vi "Power Peak Calibration.vi"() -> ()   [LabVIEW 2013]
uses:
  <vilib>/Analysis/NI_AALPro.lvlib
panel:
  in  "Acquire Data":bool
  out "df":dbl
  out "Calibration Data":dbl[](array[numeric])
  in  "Record Power Peak":bool
  out "Power Peak (V_{rms}^2)":dbl
  out "Spectrum Plot":cluster{dbl, "df":dbl, "Spectrum out":dbl[]}(graph)={0.0, "df"=976.5625, "Spectrum out"=[-15.845905781941731, -43.915142224307615, -49.190152957598016, -53.852042141976526, -56.401103239588394, -57.085019943821614, -57.42779024840779, -57.35398394101817, -56.62922799689663, -55.89570951726039, -56.17500389904336, -56.658091219147195, -57.96434809011062, -59.59705407171775, -60.67339237533791, -61.360791233190774, -62.26267752184724, -63.423104999089006, -63.73866172675654, -64.18018519332178, -64.68423775328336, -64.98272548894641, -64.65310396761447, -64.57730161736126, -64.6005007874894, -64.12943876516434, -64.40965139054964, -64.48190909962165, -64.18589412754218, -64.42687756848638, -64.73568364963023, -65.28016436445176, -65.51147244197554, -65.98403978636362, -66.34146853538246, -66.55039985238902, -67.06053323082511, -67.74164293441598, -67.93985420802743, -68.61366318004022, -68.72894399366066, -68.87062306002007, -69.25800759395273, -69.1836018440649, -69.6828981066074, -70.13235629974473, -70.02165546204415, -70.33805295925532, -70.33684508822006, -70.7747643357369, -70.92095605059647, -70.96159422425444, -71.51578558675507, -71.41022976627563, -71.51054007786686, -71.70594752739161, -71.89852623371247, -72.25001369052693, -72.05827807939693, -72.39722220210967, -72.26810938379876, -72.41633072401957, -72.89508447023017, -72.99611346447384, -72.86737450753068, -73.0319650267352, -73.4268723195781, -73.65485289175722, -73.76856016219259, -74.38259001523501, -74.49537543116152, -74.74289986108654, -74.52927345921171, -74.90899995658931, -75.12881029655497, -75.14682651299673, -76.04632955612527, -75.94928207346015, -75.99537357070861, -76.4528123167457, -76.58018971613478, -76.85262666813362, -76.94211368376116, -77.18033274801466, -77.34416946182976, -77.97653501905563, -78.08882898139076, -77.75504318146395, -78.61320071718298, -78.70255681878588, -78.89431147000928, -79.14802147917631, -79.24488934190079, -79.65778031243343, -79.75057207068667, -79.77429060312991, -80.22466006530694, -80.68765140609128, -80.74976372106957, -81.0940546603702, -81.06408506915871, -81.82084451213092, -81.88988589649128, -81.84353327749841, -82.71246581831555, -82.51089752593228, -82.76564863813098, -83.37330766537886, -83.57000868373369, -84.207392955926, -83.969059548894, -83.78119345015493, -84.68397306775822, -85.0123761871565, -85.04032792293864, -85.23566564306427, -85.49339332769287, -86.10740873526836, -86.30750461634167, -86.4954000769498, -86.58840326479293, -86.89617522722962, -87.03534322616281, -87.46765008133713, -87.51609655554547, -88.10480512426382, -88.53915071524821, -88.19089444702308, -88.76142323860263, -88.71484736501934, -89.39078167881094, -89.1390929539335, -89.73983451982647, -89.43411209172332, -90.07683547720683, -89.84084792738655, -90.03935645658841, -90.50074846778033, -90.62364106944639, -90.51858213646457, -90.77967673354854, -90.93487931797472, -90.49480094125931, -90.3356032916364, -91.24246400073463, -91.48972525529442, -91.56992962340016, -91.76393867194281, -92.24132938539142, -91.75033976436218, -92.23161782472576, -87.81832550071526, -91.95848559189331, -92.41846454494608, -92.44911534680506, -92.40717315350687, -92.64568182466519, -92.57261319696957, -92.68207058954437, -92.9414768787689, -92.99508291320579, -92.867293420003, -92.94829912779514, -93.22977946462234, -93.1496226108207, -93.32130652503764, -93.23714576357534, -92.71904125124473, -93.18861501311126, -93.34592185157314, -93.45645354610178, -93.29578779965661, -93.3961297071871, -93.52984447013718, -92.02818183792024, -92.17337335281373, -93.28573212068224, -93.4340403695752, -93.84898362415335, -93.8581389607782, -93.89732009520142, -93.8717074429978, -93.55264052897613, -93.50847613972101, -94.08331357574471, -94.07085225312551, -94.12661608080454, -94.3287445314006, -94.21766199449495, -94.27011202232808, -93.74524014468926, -94.35069940715115, -94.57610154940247, -94.52140154491451, -94.506512103288, -94.56804830787351, -94.49032013599088, -94.46360025059532, -94.28632692138267, -94.49959977802484, -94.50646018472031, -94.40554926428291, -94.68078780859665, -94.64664127985617, -94.66194886677796, -94.47957139621263, -93.31930218448838, -91.90550929382852, -94.34111457198259, -94.68074039683111, -94.79277504034081, -94.67994321030025, -94.86846988585798, -94.59982729948628, -94.07756932717759, -93.94330857800993, -94.30027374612484, -94.96329133863675, -94.77334352200275, -95.17028193906157, -95.21627296027212, -94.89033645488158, -95.20261401452001, -94.7704132670353, -95.42628192610192, -95.15102974391041, -95.18733765508992, -95.14908122444831, -95.4464140437162, -95.42528161153442, -94.48555734817637, -95.1993983585333, -95.39889184869536, -95.4903325691213, -95.48979359017684, -95.48200245883402, -95.49936365987897, -95.24916272786852, -91.91217566611354, -94.47496647183172, -95.27773576498515, -95.62838774635402, -95.71895141030696, -95.88390829882444, -95.56255178116972, -95.56813843723248, -95.07076550467647, -95.41001727617747, -95.58615607679087, -95.74834461273437, -95.77760596931367, -95.97902444733214, -95.94618628531285, -96.125407389205, -96.05556462687056, -95.63456098032873, -95.85612018930411, -95.80426046264252, -95.85838083397036, -95.70135694128692, -95.92486020964407, -95.77151462988817, -95.56348235993723, -95.63278256966903, -95.92343511351353, -95.84676472701682, -95.98333279604728, -96.25747326594166, -95.91741144469422, -95.36123720048207, -93.53184100084428, -95.92088328158893, -95.67059250119598, -96.08314273525487, -96.08815002286863, -96.22857738603786, -95.79857795122776, -95.73640081941579, -87.83199015388689, -95.89330062152945, -96.38888519003386, -96.39583952467083, -96.48390492192655, -96.61453120154768, -96.67350640699806, -96.56146072576644, -96.27150366452624, -96.59490502386653, -96.42327820826156, -96.49183302613625, -96.53913950676514, -96.49314016260925, -96.23812751552953, -95.8866021994261, -95.54556448224449, -96.45802589344208, -96.7081588901148, -96.34268723583261, -96.5775070247212, -96.0158615492137, -95.60991718375256, -92.98295890874621, -93.1175643950674, -95.48928276599159, -96.22343360123936, -96.58719806894042, -96.25366695891285, -96.70869216556476, -96.75664104310033, -95.99058593639634, -94.64288633299653, -96.39354296370634, -96.72512038071808, -96.89323897924083, -97.16294983631505, -96.99550829692208, -97.07580684762681, -97.05727223406919, -96.81028630212607, -97.00924445063612, -96.93954724005931, -96.910905559072, -97.25053999912566, -97.09809186624064, -96.99480693304544, -96.75674825164693, -96.71418496792745, -97.01481312025051, -96.98148452558607, -97.01830796226021, -96.69339813471524, -96.59361393554506, -96.4309846912819, -94.38407178672736, -92.50436488753007, -96.01557282796318, -96.39356474689868, -97.01610959436871, -97.05636935662201, -96.94226548253532, -96.0803835936364, -94.55887738493533, -94.20134587085661, -95.49518187885134, -96.66382783262259, -96.86250971219577, -97.00560385732297, -96.96730073141048, -97.0953639128831, -96.89780822210325, -96.48712240274082, -96.7856155647513, -96.72125010071417, -96.58394972410399, -96.6221299103751, -96.66884759315269, -96.73433925619264, -96.33613482351356, -96.89289999301926, -96.03898417460942, -97.09920512469947, -96.97039713471543, -96.67214133783074, -96.78650672809556, -95.9112797853549, -88.64340678313235, -95.24547674087896, -96.68477510092077, -97.26506755337493, -97.1141231148176, -97.2139546520637, -97.30526535922769, -97.18621986933206, -94.2064163293791, -96.39143663947267, -97.2802323889613, -97.54892117980299, -97.36965609295105, -97.26059900417418, -97.11769961105392, -96.61078438140439, -97.23469909611896, -97.7011904395048, -97.39540003198924, -97.31676145868914, -97.49636186951997, -97.19736596978883, -97.06772766971199, -96.63770097352807, -96.53253764690933, -96.24702084266804, -96.41431118366324, -96.0911845626953, -95.83696385570606, -95.78547289086474, -95.20587090233619, -94.14965366487957, -91.98394335062423, -94.42258288009647, -94.86573505676839, -95.20179207612364, -95.78589887823911, -96.02483899744861, -96.3232417400719, -94.37664270069325, -84.63776042475754, -95.90833150645543, -96.85168271545405, -96.94917553463841, -97.25201393296331, -97.19803469804113, -97.44067231757063, -97.28856434493133, -96.28089076443857, -97.40157405797581, -97.29153510147472, -97.60517422678114, -97.57431936262054, -97.3721504279831, -97.53879903587708, -96.19909166372716, -96.25534829018159, -97.09750465448909, -97.00543625791937, -97.15095351396809, -96.58677119756445, -95.86194320630636, -93.96685771994126, -90.41654167200038, -91.0693693812922, -94.9513584929577, -96.28027049834664, -96.94590502670485, -96.94649852135676, -96.93113649614565, -96.56082193420788, -95.07817706510154, -93.86060076780025, -96.52071349387154, -97.21608851333141, -97.41488438212835, -97.46100333688378, -97.54199390581512, -97.58802567652239, -97.73748653957938, -97.41143723707317, -97.64500942619026, -97.74567328179786, -97.31304599093758, -97.68415263166796, -97.47817511849203, -97.48054466789846, -97.04145721392551, -97.13368056999023, -97.02339838743785, -97.32646604511258, -97.29690558109404, -97.39432260133225, -96.5389671686748, -96.36745891004183, -93.32306114208308, -93.52279253865957, -96.06301720725452, -96.99679379652507, -97.22296553195883, -96.7803464077598, -96.17262512321993, -94.41741314352049, -90.69349735405582, -90.30864158287707, -93.60468105114984, -95.72116646020368, -96.72892404876248, -97.29206802349279, -97.33409428132504, -96.89003477779283, -96.65097311154193, -95.67336679796946, -97.35096090415384, -97.73586554491067, -97.37883119018427, -97.21263091086533, -97.2512543565889, -96.74699835373269, -95.8191731459854, -96.00648696385674, -96.52816706888403, -96.09462064468252, -95.71864506376434, -95.36446930336453, -94.5220549369676, -94.28861575473039, -82.41886951077308, -92.57965888998464, -95.25193795443043, -95.85967031154053, -96.36845271373369, -96.76148137360579, -96.64203396550224, -95.85239753081248, -90.57107701319113, -94.67355653996842, -96.74735861289072, -97.27384173670609, -97.52510444563741, -97.44490997000153, -97.79406408672072, -96.89645362371891, -97.16653693392722, -97.48342716272393, -97.75527760586351, -97.77211964146444]}
  # "Acquiring Data..."
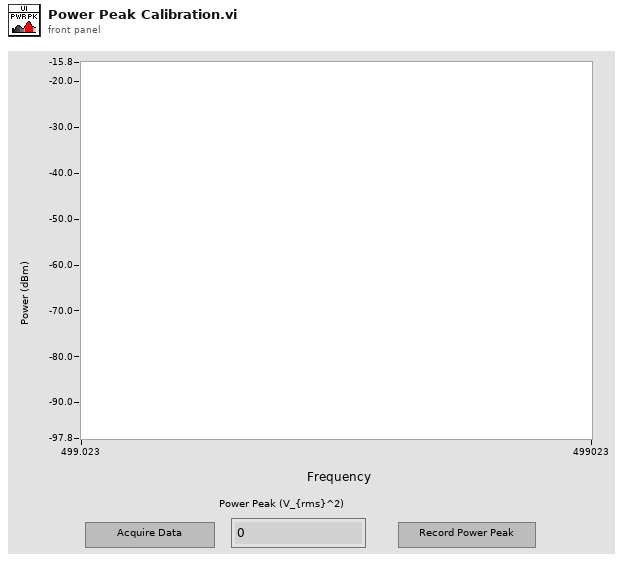
[diagram p1: front panel]
types:
  T1 = enum32{"Vrms", "Vpk", "Vrms^2", "Vpk^2", "Vrms/rtHz", "Vpk/rtHz", "Vrms^2/Hz", "Vpk^2/Hz"}
  T2 = enum16{"Power (Vrms^2)", "Amplitude (Vrms)", "Gain (amplitude ratio)"}
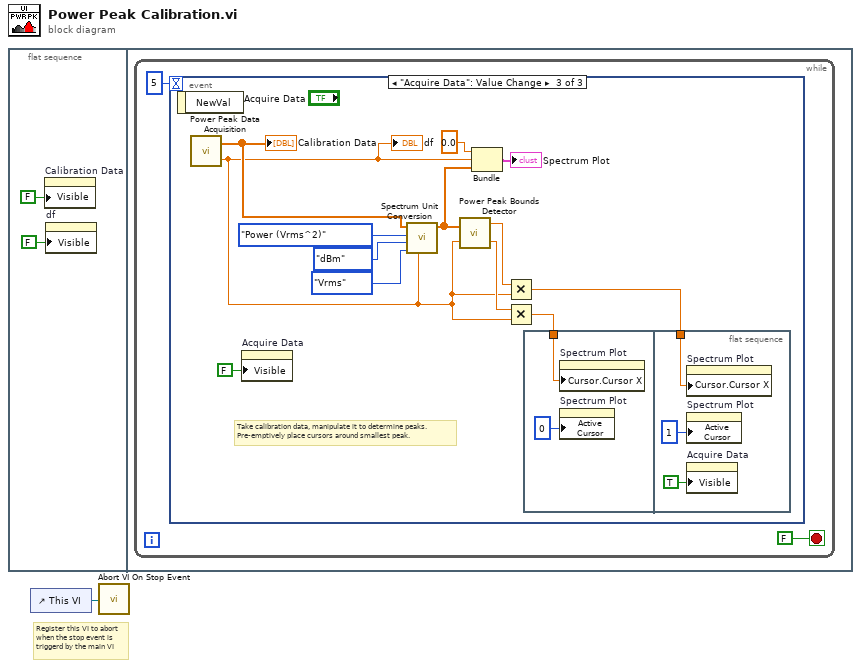
[diagram p0: block diagram]
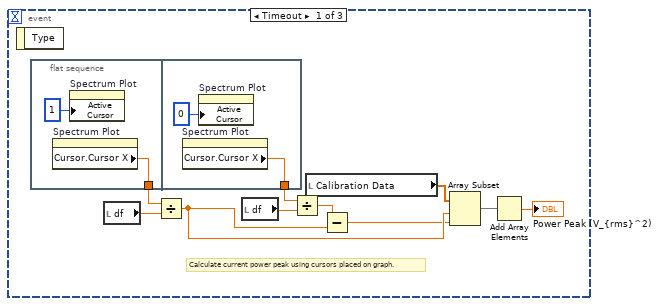
[diagram p2: hidden frame]
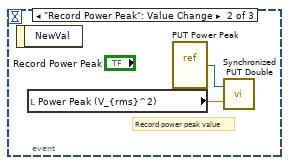
[diagram p3: hidden frame]
diagram:
  # "Register this VI to abort\nwhen the stop event is\ntriggerd by the main VI"
  n1 = flat-sequence {
    frame #0 {
      n2 = property on="Calibration Data" class="Arr (strict)"("Visible"=FALSE) -> ()  [unwired: 2 in, 2 out]
      n3 = property on="df" class="DigNum (strict)"("Visible"=FALSE) -> ()  [unwired: 2 in, 2 out]
    }
    frame #1 {
      n4 = while {
        stop <- FALSE stop-if-true
        n5 = event shown="[2] \"Acquire Data\": Value Change" {
          selector: _ -> [_ _ _]
          dyn-events: _ -> [_ _ _]
          timeout: 5 -> [_ _ _]
          event Timeout {
            # "Calculate current power peak using cursors placed on graph."
            n6 = event-data() -> ()  [unwired: 1 in, 1 out]
            n7 = flat-sequence {
              tunnel: [w16] -> w12
              tunnel: [w18] -> w14
              frame #0 {
                n8 = property on="Spectrum Plot" class="WFGraph (strict)"() -> ("Cursor.Cursor X"=w16:dbl)  [unwired: 2 in, 2 out]
                n9 = property on="Spectrum Plot" class="WFGraph (strict)"("Active Cursor"=u32 1) -> ()  [unwired: 2 in, 2 out]
              }
              frame #1 {
                n10 = property on="Spectrum Plot" class="WFGraph (strict)"() -> ("Cursor.Cursor X"=w18:dbl)  [unwired: 2 in, 2 out]
                n11 = property on="Spectrum Plot" class="WFGraph (strict)"("Active Cursor"=u32 0) -> ()  [unwired: 2 in, 2 out]
              }
            }
            n12 = local read "df"() -> (w8:dbl)
            n13 = Divide(x=w12, y=w8) -> (x/y=w15:dbl)
            n14 = local read "df"() -> (w6:dbl)
            n15 = Divide(x=w14, y=w6) -> (x/y=w13:dbl)
            n16 = local read "Calibration Data"() -> (w7:dbl[])
            n17 = Subtract(x=w13, y=w15) -> (x-y=w11:dbl)
            n18 = Array Subset(array=w7, index=w15, length=w11) -> (w10:dbl[])
            n19 = Add Array Elements(numeric array=w10) -> (sum=→"Power Peak (V_{rms}^2)":dbl)
          }
          event "Record Power Peak": Value Change {
            # "Record power peak value"
            n20 = event-data() -> ()  [unwired: 1 in, 1 out]
            n21 = local read "Power Peak (V_{rms}^2)"() -> (w20:dbl)
            n22 = vi-ref "PUT Power Peak.vi"() -> (w21:refnum<vi>)
            n23 = call "Synchronized PUT Double.vi"("PUT Value"=w20, "PUT VI Reference"=w21) -> ()  [unwired: 1 in]
          }
          event "Acquire Data": Value Change {
            # "Take calibration data, manipulate it to determine peaks.\nPre-emptively place cursors around smallest peak."
            n24 = event-data() -> ()  [unwired: 1 in, 1 out]
            n25 = call "Power Peak Data Acquisition.vi"() -> ("df"=w24:dbl, "Calibration Data"=w25:dbl[])  [unwired: 2 in]
            "Calibration Data" <- w25
            "df" <- w24
            n26 = property on="Acquire Data" class="Bool"("Visible"=FALSE) -> ()  [unwired: 2 in, 2 out]
            n27 = call <vilib>:"Spectrum Unit Conversion.vi"("df"=w24, "display unit"=T1."Vrms", "log/linear"=enum16{"Linear", "dB", "dBm"}."dBm", "spectrum type"=T2."Power (Vrms^2)", "Spectrum in"=w25) -> ("Spectrum out"=w30:dbl[])  [unwired: 5 in, 1 out]
            n28 = call "Power Peak Bounds Detector.vi"("df"=w24, "Signal In"=w30) -> ("min"=w28:dbl, "max"=w29:dbl)
            n29 = Bundle(0.0, "df"=w24, "Spectrum out"=w30) -> (→"Spectrum Plot":cluster{dbl, "df":dbl, "Spectrum out":dbl[]})  [unwired: 1 in]
            n30 = Multiply(x=w29, y=w24) -> (x*y=w27:dbl)
            n31 = Multiply(x=w28, y=w24) -> (x*y=w26:dbl)
            n32 = flat-sequence {
              tunnel: w26 -> [w35]
              tunnel: w27 -> [w38]
              frame #0 {
                n33 = property on="Spectrum Plot" class="WFGraph (strict)"("Cursor.Cursor X"=w35) -> ()  [unwired: 2 in, 2 out]
                n34 = property on="Spectrum Plot" class="WFGraph (strict)"("Active Cursor"=u32 0) -> ()  [unwired: 2 in, 2 out]
              }
              frame #1 {
                n35 = property on="Spectrum Plot" class="WFGraph (strict)"("Cursor.Cursor X"=w38) -> ()  [unwired: 2 in, 2 out]
                n36 = property on="Spectrum Plot" class="WFGraph (strict)"("Active Cursor"=u32 1) -> ()  [unwired: 2 in, 2 out]
                n37 = property on="Acquire Data" class="Bool"("Visible"=TRUE) -> ()  [unwired: 2 in, 2 out]
              }
            }
          }
        }
      }
    }
  }
  n38 = control-ref of="This VI"() -> (w1:refnum<vi>)
  n39 = call "Abort VI On Stop Event.vi"("VI Reference"=w1) -> ()
